vi "12_Bit_Array_To_Byte_Array.vi"(1 "12-Bit-Array":u16[](array[numeric])) -> (0 "Byte-Array":u8[](array[numeric]))   [LabVIEW 2013]
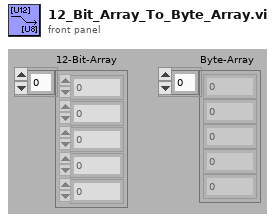
[diagram p1: front panel]
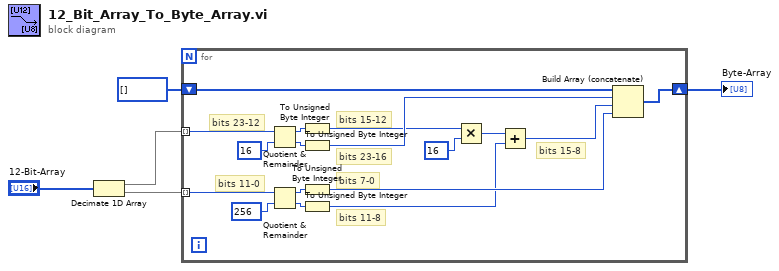
[diagram p0: block diagram]
diagram:
  n1 = Decimate 1D Array("12-Bit-Array") -> (w5:u16[], w4:u16[])
  n2 = for {
    tunnel: w5 -> [w20] mode=indexing
    tunnel: w4 -> [w15] mode=indexing
    shift-right: [w21] -> w1
    shift-left: u8[] [] -> [w22]
    # "bits 15-8"
    # "bits 11-8"
    # "bits 7-0"
    # "bits 15-12"
    # "bits 23-16"
    # "bits 11-0"
    # "bits 23-12"
    n3 = Quotient & Remainder(x=w20, y=u16 16) -> (x-y*floor(x/y)=w12:u16, floor(x/y)=w18:u16)
    n4 = Quotient & Remainder(x=w15, y=u16 256) -> (x-y*floor(x/y)=w14:u16, floor(x/y)=w11:u16)
    n5 = To Unsigned Byte Integer(number=w12) -> (unsigned 8bit integer=w10:u8)
    n6 = To Unsigned Byte Integer(number=w18) -> (unsigned 8bit integer=w17:u8)
    n7 = To Unsigned Byte Integer(number=w14) -> (unsigned 8bit integer=w13:u8)
    n8 = To Unsigned Byte Integer(number=w11) -> (unsigned 8bit integer=w7:u8)
    n9 = Multiply(x=w10, y=u8 16) -> (x*y=w8:u8)
    n10 = Add(x=w8, y=w7) -> (x+y=w6:u8)
    n11 = Build Array (concatenate)(w22, w17, w6, w13) -> (w21:u8[])
  }
  "Byte-Array" <- w1
